vi "__FilterSet_IDBtnChange.vi"(8 "error in (no error)":errorcluster, 11 "Btn Ref":refnum<vi>) -> (0 "error out":errorcluster)   [LabVIEW 2011]
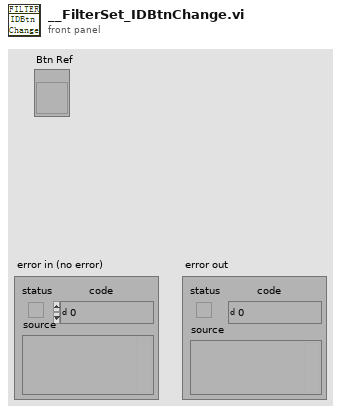
[diagram p1: front panel]
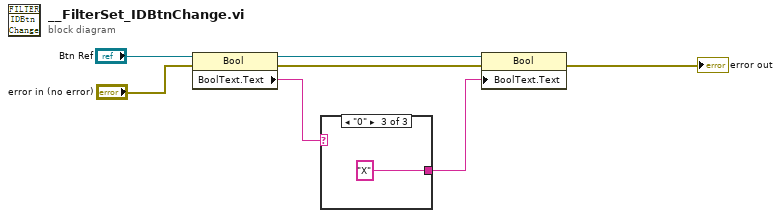
[diagram p0: block diagram]
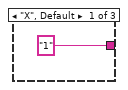
[diagram p2: hidden frame]
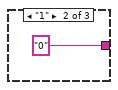
[diagram p3: hidden frame]
diagram:
  n1 = property class="Bool"(reference="Btn Ref", error in="error in (no error)") -> (reference out=w4:refnum<vi>, error out=w3:errorcluster, "BoolText.Text"=w5:string)
  n2 = case shown="\"0\"" w5 {
    tunnel: ["1" "0" "X"] -> w2
    frame "X", Default {
    }
    frame "1" {
    }
    frame "0" {
    }
  }
  n3 = property class="Bool"(reference=w4, error in=w3, "BoolText.Text"=w2) -> (error out=→"error out":errorcluster)  [unwired: 1 out]
